vi "Set V3 (SubVI).vi"(11 "Voltage Z":string) -> (3 "String":string)   [LabVIEW 2018]
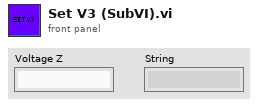
[diagram p1: front panel]
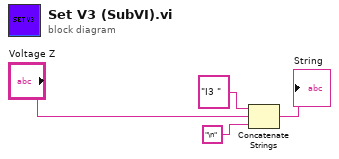
[diagram p0: block diagram]
diagram:
  n1 = Concatenate Strings("I3 ", "Voltage Z", "\n") -> (→"String":string)
